vi "dfd_FXP_Simulation_Template.vi"(5 "input range":dbl=1.0, 7 "init? (T)":bool=TRUE, 8 "error in (no error)":errorcluster, 9 "filtering statistics in":T3(array[cluster]) {"statistics information"."min value" format="%.2f"; "statistics information"."max value" format="%.2f"; "Quantizer Source" items=["Coefficients a/k"=0, "Coefficients b/v"=7, "Input"=1, "Output"=2, "Multiplicand"=3, "Product"=4, "Sum"=5, "Delay"=6]}, 10 "filter in":T4 {"mSRate_QSettings"."source" items=["Coef a/k"=0, "Coef b/v"=7, "Input"=1, "Output"=2, "Multiplicand"=3, "Product"=4, "Sum"=5, "Delay"=6, "Gain"=8]}, 11 "signal in":fxp<+/-,53,1>[](array[numeric])) -> (0 "error out":errorcluster, 1 "filtering statistics report":T3(array[cluster]) {"statistics information"."min value" format="%.2f"; "statistics information"."max value" format="%.2f"; "Quantizer Source" items=["Coefficients a/k"=0, "Coefficients b/v"=7, "Input"=1, "Output"=2, "Multiplicand"=3, "Product"=4, "Sum"=5, "Delay"=6]}, 2 "integer signal out":i32[](array[numeric]), 3 "DBL signal out":dbl[](array[numeric]))   [LabVIEW 2017]
uses:
  <vilib>/addons/Digital Filter Design/_Objects.llb/DFD Filter Obj.ctl
  <vilib>/addons/Digital Filter Design/_Objects.llb/DFD Filter Coef.ctl
  <vilib>/addons/Digital Filter Design/_Objects.llb/DFD Filter Structure Type Selector.ctl
  <vilib>/addons/Digital Filter Design/_Objects.llb/dfd_Internal Quantization Settings.ctl
  <vilib>/addons/Digital Filter Design/_Objects.llb/dfd_Internal Quantization Srcs.ctl
  <vilib>/addons/Digital Filter Design/_Objects.llb/DFD Coef Norm Type.ctl
  <vilib>/addons/Digital Filter Design/_Objects.llb/DFD Quantization Sources.ctl
  <vilib>/addons/Digital Filter Design/_Objects.llb/DFD FXP Statistics Data.ctl
  <vilib>/addons/Digital Filter Design/NI_DigFilter_FXP.lvlib
  <vilib>/Utility/VariantDataType/VariantType.lvlib
  <vilib>/addons/Digital Filter Design/NI_DigFilterLicensed.lvlib
panel:
  in  "input selector":enum16{"FXP", "Integer", "Double"}(ring)
  in  "check integer":bool
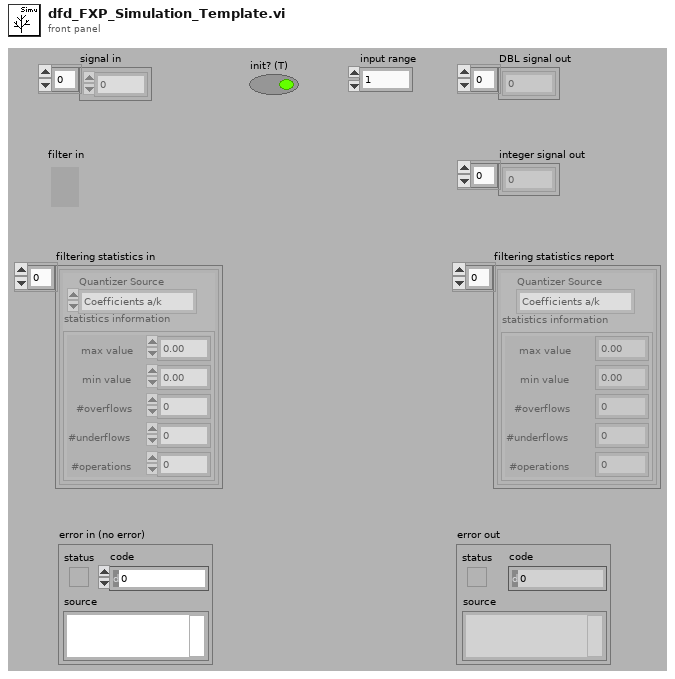
[diagram p1: front panel]
types:
  T1 = typedef "NI_DigFilterLicensed.lvlib/DFD Quantization Sources.ctl" = u16
  T2 = typedef "NI_DigFilterLicensed.lvlib/DFD FXP Statistics Data.ctl" = cluster{"max value":ext, "min value":ext, "#overflows":i32, "#underflows":i32, "#operations":i32}
  T3 = cluster{"Quantizer Source":T1, "statistics information":T2}[]
  T4 = typedef "NI_DigFilterLicensed.lvlib/DFD Filter Obj.ctl" = cluster{"mSRate_Fs":dbl, "mSRate_Version":string, "mSRate_Comments":string, "mSRate_OrgCoef":T5, "mSRate_CurCoef":T5, "mSRate_Quantized?":bool, "mSRate_QCoef":T5, "mSRate_QSettings":T7[], "mSRate_Order":i32, "mSRate_Scaling":cluster{"mSRate_ScaleByPowerOf2?":bool, "mSRate_ScaleType":T9}}
  T5 = typedef "NI_DigFilterLicensed.lvlib/DFD Filter Coef.ctl" = cluster{"type":T6, "gain":dbl, "coef a (k)":dbl[], "coef b (v)":dbl[]}
  T6 = typedef "NI_DigFilterLicensed.lvlib/DFD Filter Structure Type Selector.ctl" = enum16{"Undefined", "FIR Direct Form", "FIR Direct Form Transposed", "FIR Symmetric", "FIR Antisymmetric", "IIR Direct Form I", "IIR Direct Form I Transposed", "IIR Direct Form II", "IIR Direct Form II Transposed", "IIR Cascaded Second Order Sections Form I", "IIR Cascaded Second Order Sections Form I Transposed", "IIR Cascaded Second Order Sections Form II", "IIR Cascaded Second Order Sections Form II Transposed", "Lattice Allpass (basic sections)", "Lattice Allpass (one multiplier sections)", "Lattice Allpass (normalized sections)", "Lattice AR (basic sections)", "Lattice AR (one multiplier sections)", "Lattice AR (normalized sections)", "Lattice MA (minimum phase)", "Lattice MA (maximum phase)", "Lattice ARMA (basic sections)", "Lattice ARMA (one multiplier sections)", "Lattice ARMA (normalized sections)"}
  T7 = typedef "NI_DigFilterLicensed.lvlib/dfd_Internal Quantization Settings.ctl" = cluster{"source":T8, "wl":i16, "iwl":i16, "overflow mode":enum16{"Saturation", "Wrap"}, "rounding mode":enum16{"Nearest", "Truncation"}, "signed?":bool}
  T8 = typedef "NI_DigFilterLicensed.lvlib/dfd_Internal Quantization Srcs.ctl" = u16
  T9 = typedef "NI_DigFilterLicensed.lvlib/DFD Coef Norm Type.ctl" = enum16{"No Norm", "Time Domain 1-Norm", "Time Domain 2-Norm", "Time Domain Inf-Norm"}
  T10 = typedef "LVFixedPointRepBitsTypeDef.ctl" = cluster{"Signed":bool, "Word Length":u32, "Integer Word Length":i32}
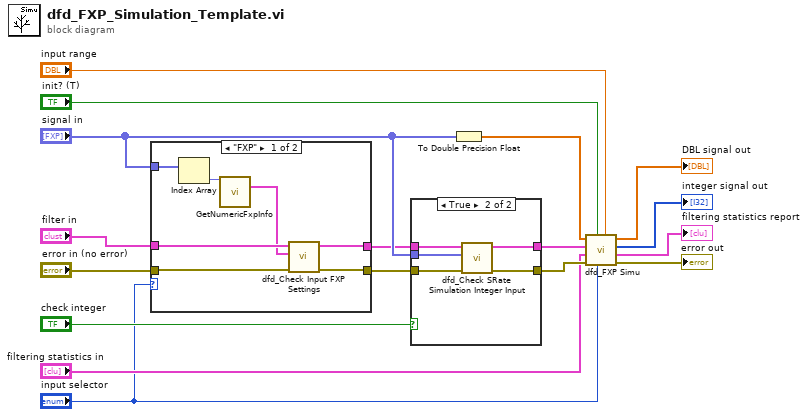
[diagram p0: block diagram]
diagram:
  n1 = case shown="\"FXP\"" "input selector" {
    tunnel: "error in (no error)" -> [w22 w26]
    tunnel: [w21 w26] -> w4
    tunnel: "filter in" -> [w19 w25]
    tunnel: "signal in" -> [w24 _]
    tunnel: [w20 w25] -> w1
    frame "FXP" {
      n2 = Index Array(array=w24) -> (element=w23:fxp<+/-,53,1>)  [unwired: 1 in]
      n3 = call <vilib>:"GetNumericFxpInfo.vi"("Variant"=w23) -> ("FxpRepresentation"=w18:T10)  [unwired: 1 in, 13 out]
      n4 = call <vilib>:"dfd_Check Input FXP Settings.vi"("error in (no error)"=w22, "FxpRepresentation"=w18, "filter in"=w19) -> ("error out"=w21:errorcluster, "filter out"=w20:T4)  [unwired: 7 out]
    }
    frame "Integer", Default {
    }
  }
  n5 = case shown="True" "check integer" {
    tunnel: w1 -> [w28 w33]
    tunnel: [w28 w32] -> w14
    tunnel: w4 -> [w27 w31]
    tunnel: [w27 w30] -> w16
    tunnel: "signal in" -> [_ w29]
    frame False {
    }
    frame True {
      n6 = call <vilib>:"dfd_Check SRate Simulation Integer Input.vi"("error in (no error)"=w31, "signal in"=w29, "filter"=w33) -> ("error out"=w30:errorcluster, "dup multirate filter"=w32:T4)  [unwired: 7 out]
    }
  }
  n7 = To Double Precision Float(number="signal in") -> (double precision float=w15:dbl[])
  n8 = call <vilib>:"dfd_FXP Simu.vi"("input range"="input range", "input selector"="input selector", "init? (T)"="init? (T)", "error in (no error)"=w16, "filtering statistics in"="filtering statistics in", "filter"=w14, "signal in"=w15) -> ("error out"=→"error out":errorcluster, "filtering statistics out"=→"filtering statistics report":T3, "integer signal out"=→"integer signal out":i32[], "DBL signal out"=→"DBL signal out":dbl[])  [unwired: 1 out]
